vi "DistributeControls.vi"(8 "error in (no error)":errorcluster, 10 "override item array":T1[](array[typedef]), 11 "VI reference":refnum<vi>) -> (0 "error out":errorcluster, 3 "VI reference out":refnum<vi>, 4 "ordered parents not found":string[](array[string]), 6 "ordered items not found":string[](array[string]))   [LabVIEW 2020, in "verticalDistribution.lvlib"]
doc: "The VI will vertically distribute all visible front panel controls (excluding free labels and decorations!), inserting a set vertical space (number of pixels) that is appropriate for all platforms. This is akin to using LabVIEW's Distribute tool with the Vertical Gap option. Extra space is added before each Section control. \n\nIf two or more controls need to be horizontally aligned, use the Ordered item array. This allows for explicit item-parent coupling. Specify item-parent relationships in a top-down order so that items that are also parents to other items are specified first. When there are two or more controls that are horizontally aligned, care needs to be taken for vertical collisions. This VI will check for collisions prior to start of new section and set section top to be below all control bottoms."
uses:
  <vilib>/Utility/vertDist/verticalDistribution.lvlib
  <vilib>/Utility/vertDist/ItemParentCtl.ctl
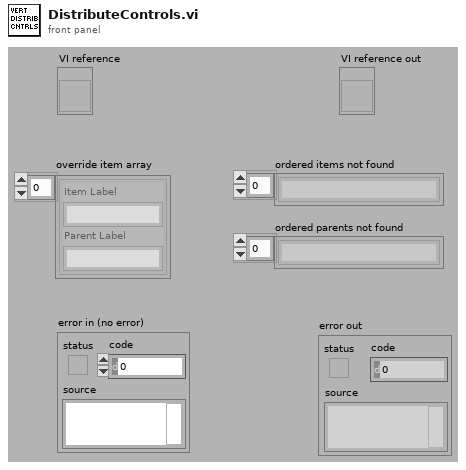
[diagram p1: front panel]
types:
  T1 = typedef "verticalDistribution.lvlib/ItemParentCtl.ctl" = cluster{"Item Label":string, "Parent Label":string}
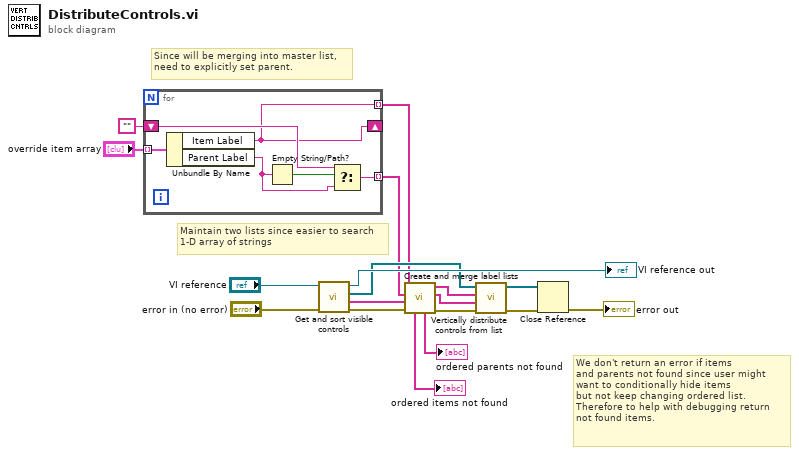
[diagram p0: block diagram]
diagram:
  # "Maintain two lists since easier to search\n1-D array of strings"
  # "Since will be merging into master list,\nneed to explicitly set parent."
  # "We don't return an error if items\nand parents not found since user might\nwant to conditionally hide items \nbut not keep changing ordered list.\nTherefore to help with debugging return\nnot found items."
  n1 = for {
    shift-right: [w19] -> _
    shift-left: "" -> [w23]
    tunnel: "override item array" -> [w21] mode=indexing
    tunnel: [w20] -> w4 mode=indexing
    tunnel: [w19] -> w3 mode=indexing
    n2 = Unbundle By Name(w21) -> ("Item Label"=w19:string, "Parent Label"=w22:string)
    n3 = Empty String/Path?(string/path=w22) -> (empty?=w24:bool)
    n4 = Select(t=w23, s=w24, f=w22) -> (s? t:f=w20:string)
  }
  n5 = call <vilib>:"Get and sort visible controls.vi"("error in (no error)"="error in (no error)", "VI reference"="VI reference") -> ("error out"=w17:errorcluster, "Ordered control labels"=w7:string[], "Visible control references"=w8:refnum<vi>[], "VI reference out"=→"VI reference out":refnum<vi>)  [unwired: 6 out]
  n6 = call <vilib>:"Create and merge label lists.vi"("error in (no error)"=w17, "Ordered item labels"=w7, "Override parent list"=w4, "Override item list"=w3) -> ("error out"=w16:errorcluster, "Merged parent list"=w1:string[], "Merged item list"=w2:string[], "ordered parents not found"=→"ordered parents not found":string[], "ordered items not found"=→"ordered items not found":string[])  [unwired: 3 out]
  n7 = call <vilib>:"Vertically distribute controls from list.vi"("error in"=w16, "Ordered parent labels"=w1, "Ordered item labels"=w2, "Sorted control references in"=w8) -> ("error out"=w14:errorcluster, "Sorted control references out"=w12:refnum<vi>[])  [unwired: 6 out]
  n8 = Close Reference(reference=w12, error in (no error)=w14) -> (error out=→"error out":errorcluster)
